vi "Get DriveTrain Encoder.vi"() -> ()   [LabVIEW 2014]
panel:
  out "Right Distance":dbl
  out "Center Distance":dbl
  out "Left Distance":dbl
  out "Right Rate":dbl
  out "Center Rate":dbl
  out "Left Rate":dbl
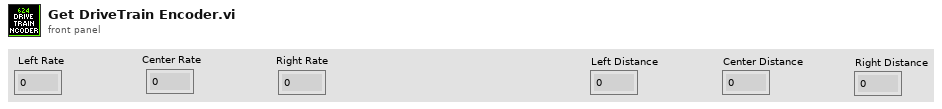
[diagram p1: front panel]
types:
  T1 = typedef "WPI_EncoderDevRef.ctl" = cluster{"DevStatus":errorcluster, "EncoderIndex":T2, "CounterIndex":T3, "DistancePerCount":dbl, "Decoding Type":T4}
  T2 = typedef "FPGA_EncoderIdx.ctl" = enum8{"Enc 0", "Enc 1", "Enc 2", "Enc 3", "Enc 4", "Enc 5", "Enc 6", "Enc 7", "Invalid"}
  T3 = typedef "FPGA_CounterCtrSystemIndex.ctl" = enum8{"Ctr 0", "Ctr 1", "Ctr 2", "Ctr 3", "Ctr 4", "Ctr 5", "Ctr 6", "Ctr 7", "Invalid"}
  T4 = typedef "WPI_EncoderType.ctl" = enum16{"1x", "2x", "4x"}
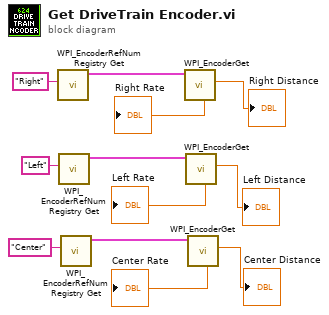
[diagram p0: block diagram]
diagram:
  n1 = call <vilib>:"WPI_EncoderRefNum Registry Get.vi"("refnum name"="Right") -> ("EncoderDevRef"=w10:T1)  [unwired: 9 in, 1 out]
  n2 = call <vilib>:"WPI_EncoderRefNum Registry Get.vi"("refnum name"="Left") -> ("EncoderDevRef"=w12:T1)  [unwired: 9 in, 1 out]
  n3 = call <vilib>:"WPI_EncoderRefNum Registry Get.vi"("refnum name"="Center") -> ("EncoderDevRef"=w8:T1)  [unwired: 9 in, 1 out]
  n4 = call <vilib>:"WPI_EncoderGet.vi"("EncoderDevRef"=w10) -> ("Distance"=→"Right Distance":dbl, "Rate"=→"Right Rate":dbl)  [unwired: 5 in, 4 out]
  n5 = call <vilib>:"WPI_EncoderGet.vi"("EncoderDevRef"=w12) -> ("Distance"=→"Left Distance":dbl, "Rate"=→"Left Rate":dbl)  [unwired: 5 in, 4 out]
  n6 = call <vilib>:"WPI_EncoderGet.vi"("EncoderDevRef"=w8) -> ("Distance"=→"Center Distance":dbl, "Rate"=→"Center Rate":dbl)  [unwired: 5 in, 4 out]
